vi "readCalib.vi"(8 "error in (no error) 2":errorcluster, 11 "Settings":T10={"CamSettings"={"Cam 0"={"position"=0.0, "pixelsize"=0.0, "start"=0.0, "end"=0.0, "center"=0.0, "Lens"=enum."FL1-f8x08", "Forward"=enum."off", "Spec_Calib_file 2"=path "Y:/100TWdata/ESMCalib/datFwd.txt", "map"=path "Y:/100TWdata/ESMCalib/mapFwd.txt", "y size"=0, "UserROI"={"Width"={"Value"=0.0, "Min"=0.0, "Max"=0.0, "StepSize"=0.0, "Tolerance"=0.0, "ValueActual"=0.0}, "Hight"={"Value"=0.0, "Min"=0.0, "Max"=0.0, "StepSize"=0.0, "Tolerance"=0.0, "ValueActual"=0.0}, "OffsetX"={"Value"=0.0, "Min"=0.0, "Max"=0.0, "StepSize"=0.0, "Tolerance"=0.0, "ValueActual"=0.0}, "OffsetY"={"Value"=0.0, "Min"=0.0, "Max"=0.0, "StepSize"=0.0, "Tolerance"=0.0, "ValueActual"=0.0}}, "CamMaxPixel"={"X"=0, "Y"=0}, "CamROI"={"Width"=0.0, "Hight"=0.0, "OffsetX"=0.0, "OffsetY"=0.0}}, "Cam 1"={"position"=0.0, "pixelsize"=0.0, "start"=0.0, "end"=0.0, "center"=0.0, "Lens"=enum."FL1-f8x08", "Forward"=enum."off", "Spec_Calib_file 2"=path "Y:/100TWdata/ESMCalib/datFwd.txt", "map"=path "Y:/100TWdata/ESMCalib/mapFwd.txt", "y size"=0, "UserROI"={"Width"={"Value"=0.0, "Min"=0.0, "Max"=0.0, "StepSize"=0.0, "Tolerance"=0.0, "ValueActual"=0.0}, "Hight"={"Value"=0.0, "Min"=0.0, "Max"=0.0, "StepSize"=0.0, "Tolerance"=0.0, "ValueActual"=0.0}, "OffsetX"={"Value"=0.0, "Min"=0.0, "Max"=0.0, "StepSize"=0.0, "Tolerance"=0.0, "ValueActual"=0.0}, "OffsetY"={"Value"=0.0, "Min"=0.0, "Max"=0.0, "StepSize"=0.0, "Tolerance"=0.0, "ValueActual"=0.0}}, "CamMaxPixel"={"X"=0, "Y"=0}, "CamROI"={"Width"=0.0, "Hight"=0.0, "OffsetX"=0.0, "OffsetY"=0.0}}, "Cam 2"={"position"=0.0, "pixelsize"=0.0, "start"=0.0, "end"=0.0, "center"=0.0, "Lens"=enum."FL1-f8x08", "Forward"=enum."off", "Spec_Calib_file 2"=path "Y:/100TWdata/ESMCalib/datFwd.txt", "map"=path "Y:/100TWdata/ESMCalib/mapFwd.txt", "y size"=0, "UserROI"={"Width"={"Value"=0.0, "Min"=0.0, "Max"=0.0, "StepSize"=0.0, "Tolerance"=0.0, "ValueActual"=0.0}, "Hight"={"Value"=0.0, "Min"=0.0, "Max"=0.0, "StepSize"=0.0, "Tolerance"=0.0, "ValueActual"=0.0}, "OffsetX"={"Value"=0.0, "Min"=0.0, "Max"=0.0, "StepSize"=0.0, "Tolerance"=0.0, "ValueActual"=0.0}, "OffsetY"={"Value"=0.0, "Min"=0.0, "Max"=0.0, "StepSize"=0.0, "Tolerance"=0.0, "ValueActual"=0.0}}, "CamMaxPixel"={"X"=0, "Y"=0}, "CamROI"={"Width"=0.0, "Hight"=0.0, "OffsetX"=0.0, "OffsetY"=0.0}}, "Cam 3"={"position"=0.0, "pixelsize"=0.0, "start"=0.0, "end"=0.0, "center"=0.0, "Lens"=enum."FL1-f8x08", "Forward"=enum."off", "Spec_Calib_file 2"=path "Y:/100TWdata/ESMCalib/datFwd.txt", "map"=path "Y:/100TWdata/ESMCalib/mapFwd.txt", "y size"=0, "UserROI"={"Width"={"Value"=0.0, "Min"=0.0, "Max"=0.0, "StepSize"=0.0, "Tolerance"=0.0, "ValueActual"=0.0}, "Hight"={"Value"=0.0, "Min"=0.0, "Max"=0.0, "StepSize"=0.0, "Tolerance"=0.0, "ValueActual"=0.0}, "OffsetX"={"Value"=0.0, "Min"=0.0, "Max"=0.0, "StepSize"=0.0, "Tolerance"=0.0, "ValueActual"=0.0}, "OffsetY"={"Value"=0.0, "Min"=0.0, "Max"=0.0, "StepSize"=0.0, "Tolerance"=0.0, "ValueActual"=0.0}}, "CamMaxPixel"={"X"=0, "Y"=0}, "CamROI"={"Width"=0.0, "Hight"=0.0, "OffsetX"=0.0, "OffsetY"=0.0}}}, "timeout"={"Value"=0.0, "Min"=0.0, "Max"=0.0, "StepSize"=0.0, "Tolerance"=0.0, "ValueActual"=0.0}, "Screws"={"Cam 0"={"S 0"={"0"=0, "1"=0, "2"=0, "3"=0}, "S 1"={"0"=0, "1"=0, "2"=0, "3"=0}, "S 2"={"0"=0, "1"=0, "2"=0, "3"=0}, "S 3"={"0"=0, "1"=0, "2"=0, "3"=0}, "S 4"={"0"=0, "1"=0, "2"=0, "3"=0}, "S 5"={"0"=0, "1"=0, "2"=0, "3"=0}}, "Cam 1"={"S 0"={"0"=0, "1"=0, "2"=0, "3"=0}, "S 1"={"0"=0, "1"=0, "2"=0, "3"=0}, "S 2"={"0"=0, "1"=0, "2"=0, "3"=0}, "S 3"={"0"=0, "1"=0, "2"=0, "3"=0}, "S 4"={"0"=0, "1"=0, "2"=0, "3"=0}, "S 5"={"0"=0, "1"=0, "2"=0, "3"=0}}, "Cam 2"={"S 0"={"0"=0, "1"=0, "2"=0, "3"=0}, "S 1"={"0"=0, "1"=0, "2"=0, "3"=0}, "S 2"={"0"=0, "1"=0, "2"=0, "3"=0}, "S 3"={"0"=0, "1"=0, "2"=0, "3"=0}, "S 4"={"0"=0, "1"=0, "2"=0, "3"=0}, "S 5"={"0"=0, "1"=0, "2"=0, "3"=0}}, "Cam 3"={"S 0"={"0"=0, "1"=0, "2"=0, "3"=0}, "S 1"={"0"=0, "1"=0, "2"=0, "3"=0}, "S 2"={"0"=0, "1"=0, "2"=0, "3"=0}, "S 3"={"0"=0, "1"=0, "2"=0, "3"=0}, "S 4"={"0"=0, "1"=0, "2"=0, "3"=0}, "S 5"={"0"=0, "1"=0, "2"=0, "3"=0}}}, "number of cam"=0.0, "X size"=0.0, "srewstart"={"Cam 0"=0.0, "Cam 1"=0.0, "Cam 2"=0.0, "Cam 3"=0.0}, "Save"=enum."off", "offset"=0.0, "localsavingpath"=path "", "ROIString"="", "exposure"={"Value"=0.0, "Min"=0.0, "Max"=0.0, "StepSize"=0.0, "Tolerance"=0.0, "ValueActual"=0.0}, "trigger"=enum."off"}) -> (0 "error out":errorcluster, 2 "fileCalib":cluster{"[0]":T1, "[1]":T1, "[2]":T1, "[3]":T1}, 3 "CamCalib":cluster{"[0]":T2, "[1]":T2, "[2]":T2, "[3]":T2}={"[0]"={"incident ANGLE COMPENSATION"=[], "dp/B [MeV/C/B]"=[], "charge compensation"=[], "Momentum [MeV/C]"=[], "energyDependence Input"=[], "pixel angle (y)"=[], "dp [MeV/C/] "=[], "angle 2Dfor spectrumj"=[], "dp [MeV/C] 2D"=[], "charge compensation 2D"=[], "Screen&Camera 2"={"Screen Orientation"="Regular", "Screen angle"="Flat", "Lens"=enum."FL1-f8x08", "Calibration (mm/pix)"=1.0}, "ROI info"={"npix-X"=0, "npix-Y"=0, "Left [pix]"=0.0, "Top [pix]"=0.0}, "Y 2D full angle"=[], "calib pixel"={"y1(pixel)"=[], "y2(pixel)"=[], "dp/B [MeV/C/B] (pixel)"=[], "energyDependence Input(pixel)"=[], "bending angle [deg](pixel)"=[], "total path(pixel)"=[], "pixel angle (y)(pixel)"=[], "energy dependence (pixel)"=[], "charge compensation (pixel)"=[], "Momentum [MeV/C](pixel)"=[], "angular compensation(pixel)"=[]}, "2D"={"dp"=[], "chargeCompensation"=[], "angle"=[], "Momentum"=[]}, "UserROI"={"Width"=0.0, "Hight"=0.0, "OffsetX"=0.0, "OffsetY"=0.0}, "final"={"X"=[], "xi"=[], "delta momentum"=0.0, "Y"=[], "yi"=[], "angle (Y)"=[], "delta angle"=0.0, "scale delta angle"=0.0, "intraX"=0.0, "intraY"=0.0, "mask"=[]}, "B[T]"=0.0, "index"=0.0}, "[1]"={"incident ANGLE COMPENSATION"=[], "dp/B [MeV/C/B]"=[], "charge compensation"=[], "Momentum [MeV/C]"=[], "energyDependence Input"=[], "pixel angle (y)"=[], "dp [MeV/C/] "=[], "angle 2Dfor spectrumj"=[], "dp [MeV/C] 2D"=[], "charge compensation 2D"=[], "Screen&Camera 2"={"Screen Orientation"="Regular", "Screen angle"="Flat", "Lens"=enum."FL1-f8x08", "Calibration (mm/pix)"=1.0}, "ROI info"={"npix-X"=0, "npix-Y"=0, "Left [pix]"=0.0, "Top [pix]"=0.0}, "Y 2D full angle"=[], "calib pixel"={"y1(pixel)"=[], "y2(pixel)"=[], "dp/B [MeV/C/B] (pixel)"=[], "energyDependence Input(pixel)"=[], "bending angle [deg](pixel)"=[], "total path(pixel)"=[], "pixel angle (y)(pixel)"=[], "energy dependence (pixel)"=[], "charge compensation (pixel)"=[], "Momentum [MeV/C](pixel)"=[], "angular compensation(pixel)"=[]}, "2D"={"dp"=[], "chargeCompensation"=[], "angle"=[], "Momentum"=[]}, "UserROI"={"Width"=0.0, "Hight"=0.0, "OffsetX"=0.0, "OffsetY"=0.0}, "final"={"X"=[], "xi"=[], "delta momentum"=0.0, "Y"=[], "yi"=[], "angle (Y)"=[], "delta angle"=0.0, "scale delta angle"=0.0, "intraX"=0.0, "intraY"=0.0, "mask"=[]}, "B[T]"=0.0, "index"=0.0}, "[2]"={"incident ANGLE COMPENSATION"=[], "dp/B [MeV/C/B]"=[], "charge compensation"=[], "Momentum [MeV/C]"=[], "energyDependence Input"=[], "pixel angle (y)"=[], "dp [MeV/C/] "=[], "angle 2Dfor spectrumj"=[], "dp [MeV/C] 2D"=[], "charge compensation 2D"=[], "Screen&Camera 2"={"Screen Orientation"="Regular", "Screen angle"="Flat", "Lens"=enum."FL1-f8x08", "Calibration (mm/pix)"=1.0}, "ROI info"={"npix-X"=0, "npix-Y"=0, "Left [pix]"=0.0, "Top [pix]"=0.0}, "Y 2D full angle"=[], "calib pixel"={"y1(pixel)"=[], "y2(pixel)"=[], "dp/B [MeV/C/B] (pixel)"=[], "energyDependence Input(pixel)"=[], "bending angle [deg](pixel)"=[], "total path(pixel)"=[], "pixel angle (y)(pixel)"=[], "energy dependence (pixel)"=[], "charge compensation (pixel)"=[], "Momentum [MeV/C](pixel)"=[], "angular compensation(pixel)"=[]}, "2D"={"dp"=[], "chargeCompensation"=[], "angle"=[], "Momentum"=[]}, "UserROI"={"Width"=0.0, "Hight"=0.0, "OffsetX"=0.0, "OffsetY"=0.0}, "final"={"X"=[], "xi"=[], "delta momentum"=0.0, "Y"=[], "yi"=[], "angle (Y)"=[], "delta angle"=0.0, "scale delta angle"=0.0, "intraX"=0.0, "intraY"=0.0, "mask"=[]}, "B[T]"=0.0, "index"=0.0}, "[3]"={"incident ANGLE COMPENSATION"=[], "dp/B [MeV/C/B]"=[], "charge compensation"=[], "Momentum [MeV/C]"=[], "energyDependence Input"=[], "pixel angle (y)"=[], "dp [MeV/C/] "=[], "angle 2Dfor spectrumj"=[], "dp [MeV/C] 2D"=[], "charge compensation 2D"=[], "Screen&Camera 2"={"Screen Orientation"="Regular", "Screen angle"="Flat", "Lens"=enum."FL1-f8x08", "Calibration (mm/pix)"=1.0}, "ROI info"={"npix-X"=0, "npix-Y"=0, "Left [pix]"=0.0, "Top [pix]"=0.0}, "Y 2D full angle"=[], "calib pixel"={"y1(pixel)"=[], "y2(pixel)"=[], "dp/B [MeV/C/B] (pixel)"=[], "energyDependence Input(pixel)"=[], "bending angle [deg](pixel)"=[], "total path(pixel)"=[], "pixel angle (y)(pixel)"=[], "energy dependence (pixel)"=[], "charge compensation (pixel)"=[], "Momentum [MeV/C](pixel)"=[], "angular compensation(pixel)"=[]}, "2D"={"dp"=[], "chargeCompensation"=[], "angle"=[], "Momentum"=[]}, "UserROI"={"Width"=0.0, "Hight"=0.0, "OffsetX"=0.0, "OffsetY"=0.0}, "final"={"X"=[], "xi"=[], "delta momentum"=0.0, "Y"=[], "yi"=[], "angle (Y)"=[], "delta angle"=0.0, "scale delta angle"=0.0, "intraX"=0.0, "intraY"=0.0, "mask"=[]}, "B[T]"=0.0, "index"=0.0}})   [LabVIEW 2020, in "MagAnalysis_Online.lvclass"]
uses:
  MagAnalysis_Online.lvclass
  MagAnalysis_Online/settings_TypDef.ctl
  CamSettings_Typdef.ctl
  CamSettingSUB_TypDEf.ctl
  CamAndObj_TypDEf.ctl
  OnOffTypeDef.ctl
  userROI.ctl
  source/Device Drivers/shared/numericVariable_TypeDef.ctl
  CamRoiTypDef.ctl
  SrewMaster_TYpDef.ctl
  srew_TypDEf.ctl
  ScrewSub_Typdef.ctl
  screwstart.ctl
  calib_Sub_Typdef.ctl
  ScreenCam2_TypDEf.ctl
  ROIInfo_TypDef.ctl
  calibPixel.ctl
  2DTypDef.ctl
  finalCalibTypdef.ctl
  configTypDEf.ctl
  specClustercommandTypdef.ctl
  source/Device Drivers/BaseDriver/BaseDriver.lvclass
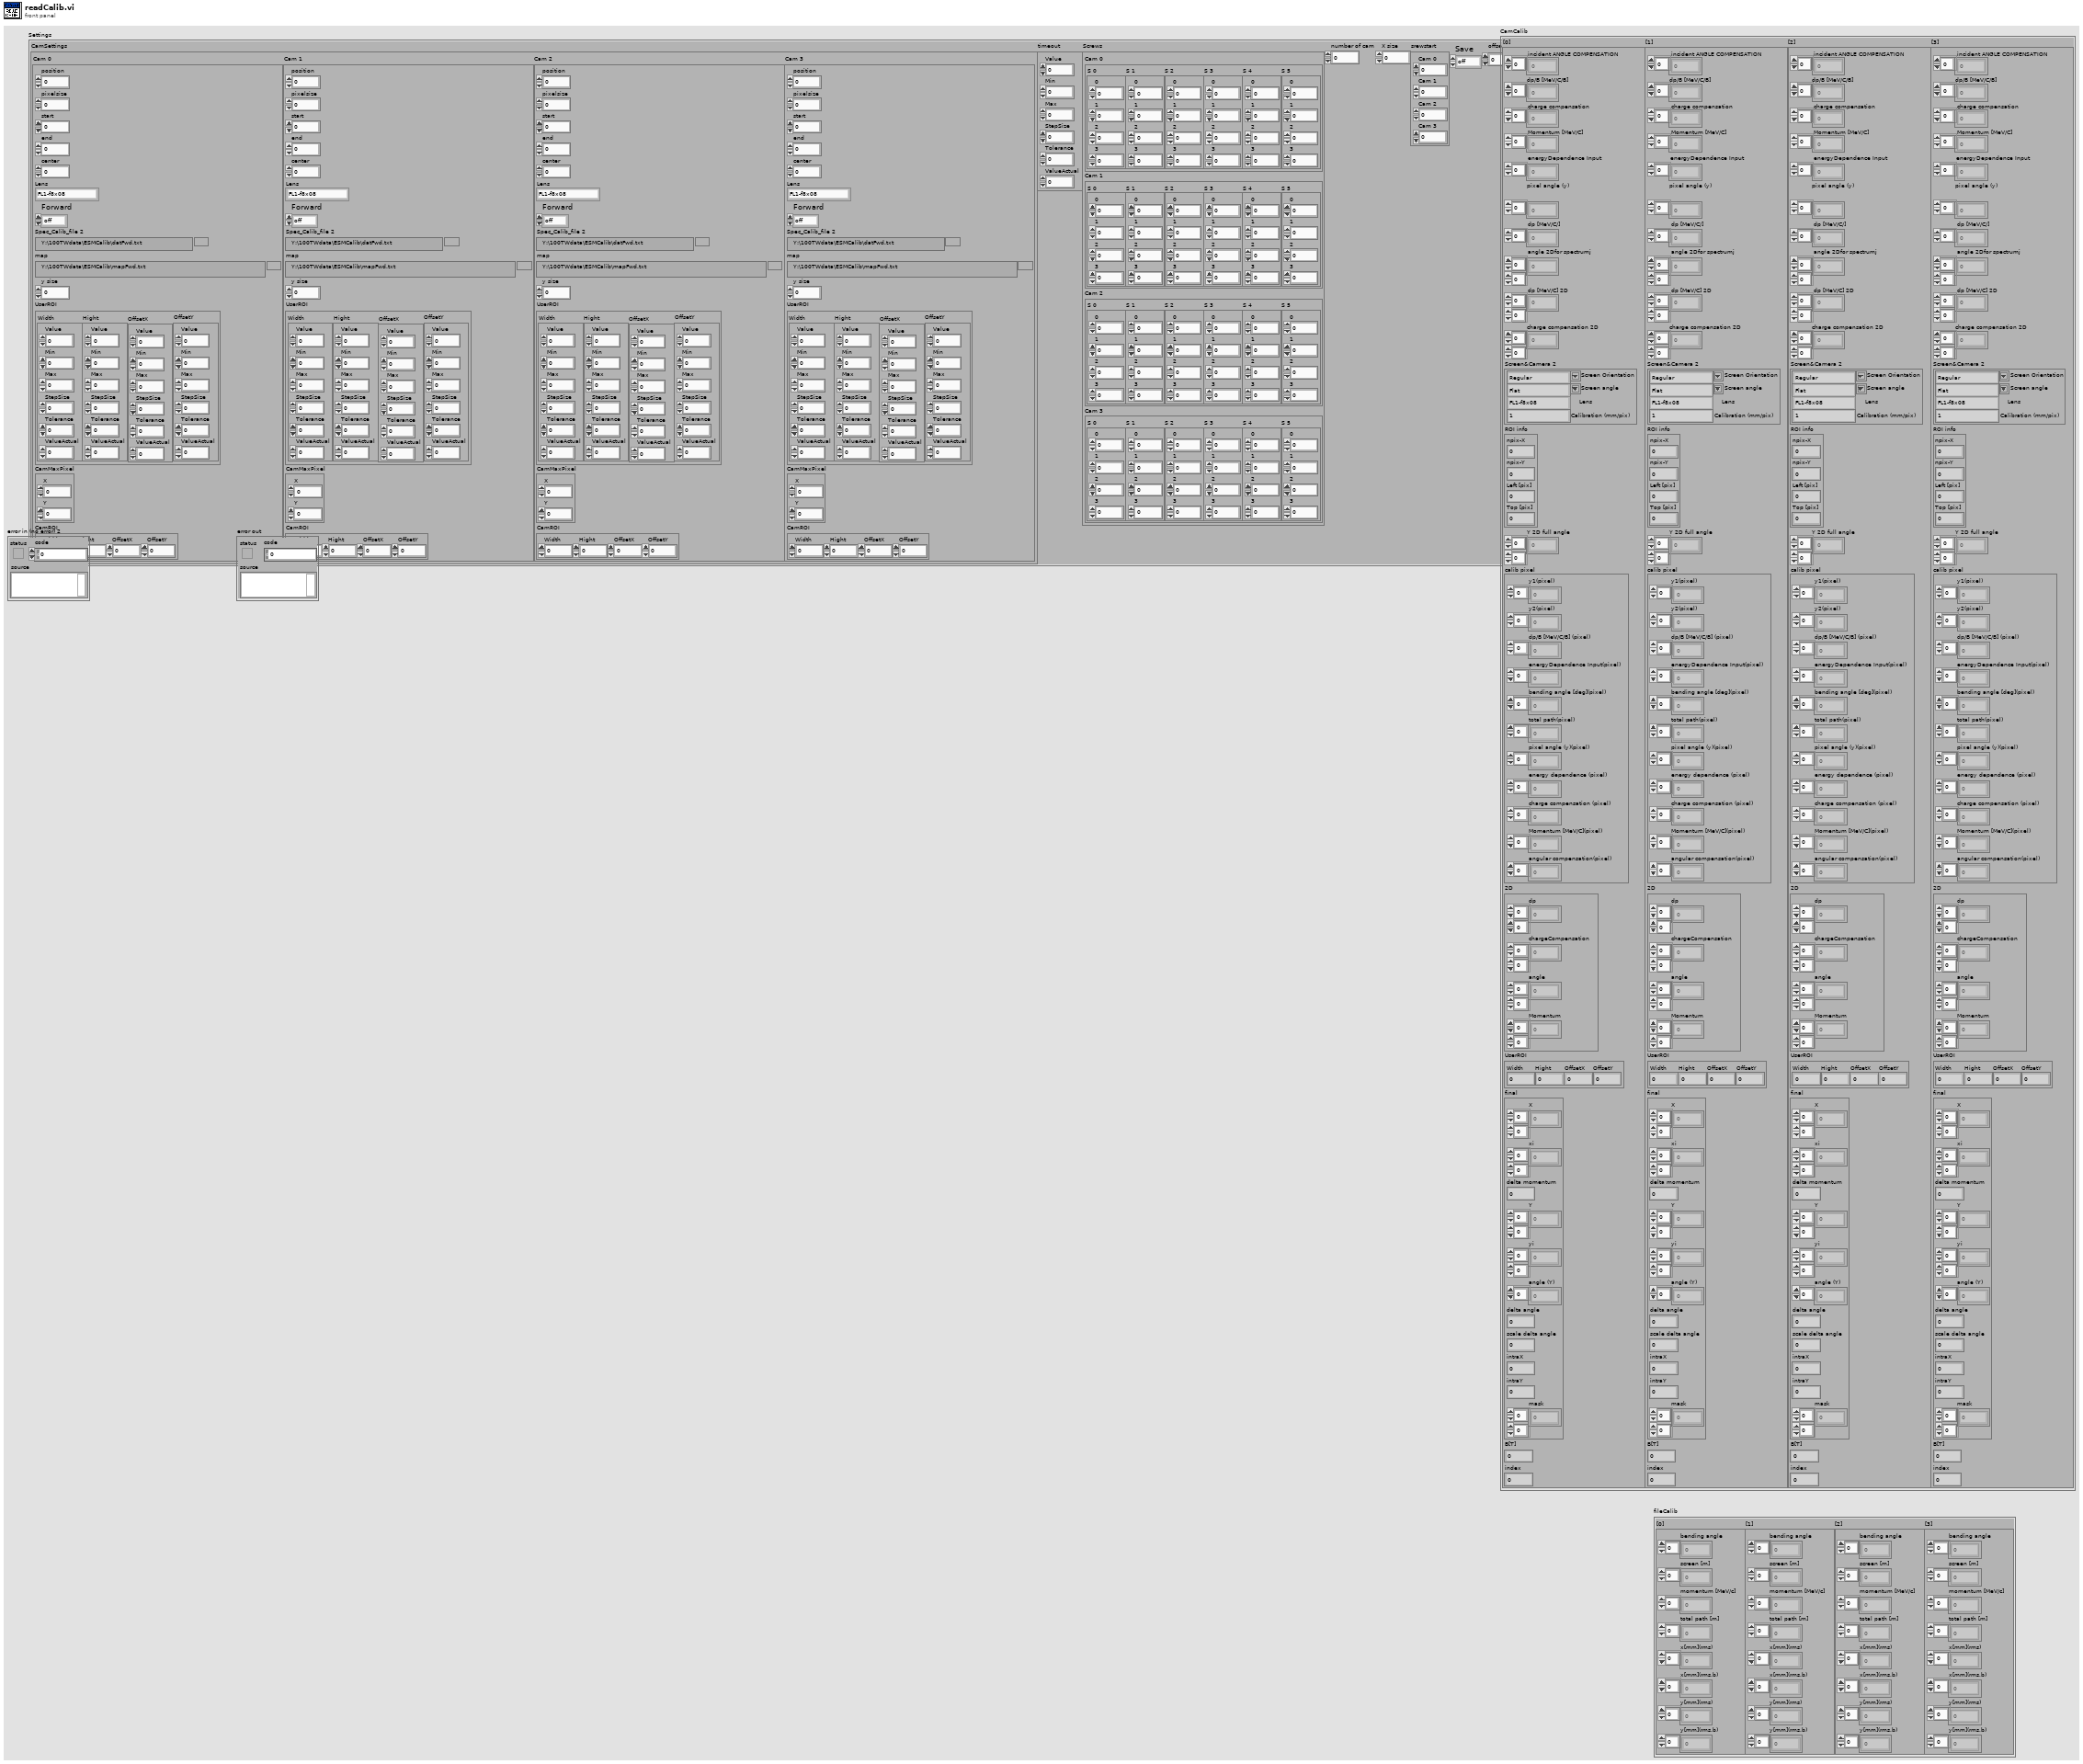
[diagram p1: front panel]
types:
  T1 = typedef "configTypDEf.ctl" = cluster{"bending angle":dbl[], "screen [m]":dbl[], "momentum [MeV/c]":dbl[], "total path [m]":dbl[], "x[mm](rms)":dbl[], "x[mm](rms,b)":dbl[], "y[mm](rms)":dbl[], "y[mm](rms,b)":dbl[]}
  T2 = typedef "calib_Sub_Typdef.ctl" = cluster{"incident ANGLE COMPENSATION":dbl[], "dp/B [MeV/C/B]":dbl[], "charge compensation":dbl[], "Momentum [MeV/C]":dbl[], "energyDependence Input":dbl[], "pixel angle (y)":dbl[], "dp [MeV/C/] ":dbl[], "angle 2Dfor spectrumj":dbl[][], "dp [MeV/C] 2D":dbl[][], "charge compensation 2D":dbl[][], "Screen&Camera 2":T3, "ROI info":T5, "Y 2D full angle":dbl[][], "calib pixel":T6, "2D":T7, "UserROI":T8, "final":T9, "B[T]":dbl, "index":dbl}
  T3 = typedef "ScreenCam2_TypDEf.ctl" = cluster{"Screen Orientation":string, "Screen angle":string, "Lens":T4, "Calibration (mm/pix)":dbl}
  T4 = typedef "CamAndObj_TypDEf.ctl" = enum16{"FL1-f8x08", "FL1-f8x06", "FL1-f8", "ch300-f50", "FL2G-f8", "FL3M14-f8", "FL3M14-f8x08", "FL3M14-f8x08(2x2)"}
  T5 = typedef "ROIInfo_TypDef.ctl" = cluster{"npix-X":i32, "npix-Y":i32, "Left [pix]":dbl, "Top [pix]":dbl}
  T6 = typedef "calibPixel.ctl" = cluster{"y1(pixel)":dbl[], "y2(pixel)":dbl[], "dp/B [MeV/C/B] (pixel)":dbl[], "energyDependence Input(pixel)":dbl[], "bending angle [deg](pixel)":dbl[], "total path(pixel)":dbl[], "pixel angle (y)(pixel)":dbl[], "energy dependence (pixel)":dbl[], "charge compensation (pixel)":dbl[], "Momentum [MeV/C](pixel)":dbl[], "angular compensation(pixel)":dbl[]}
  T7 = typedef "2DTypDef.ctl" = cluster{"dp":dbl[][], "chargeCompensation":dbl[][], "angle":dbl[][], "Momentum":dbl[][]}
  T8 = typedef "CamRoiTypDef.ctl" = cluster{"Width":dbl, "Hight":dbl, "OffsetX":dbl, "OffsetY":dbl}
  T9 = typedef "finalCalibTypdef.ctl" = cluster{"X":dbl[][], "xi":dbl[][], "delta momentum":dbl, "Y":dbl[][], "yi":dbl[][], "angle (Y)":dbl[], "delta angle":dbl, "scale delta angle":dbl, "intraX":dbl, "intraY":dbl, "mask":dbl[][]}
  T10 = typedef "MagAnalysis_Online.lvclass/settings_TypDef.ctl" = cluster{"CamSettings":T11, "timeout":T15, "Screws":T16, "number of cam":dbl, "X size":dbl, "srewstart":T19, "Save":T13, "offset":dbl, "localsavingpath":path, "ROIString":string, "exposure":T15, "trigger":T13}
  T11 = typedef "CamSettings_Typdef.ctl" = cluster{"Cam 0":T12, "Cam 1":T12, "Cam 2":T12, "Cam 3":T12}
  T12 = typedef "CamSettingSUB_TypDEf.ctl" = cluster{"position":dbl, "pixelsize":dbl, "start":dbl, "end":dbl, "center":dbl, "Lens":T4, "Forward":T13, "Spec_Calib_file 2":path, "map":path, "y size":i32, "UserROI":T14, "CamMaxPixel":cluster{"X":i32, "Y":i32}, "CamROI":T8}
  T13 = typedef "OnOffTypeDef.ctl" = enum16{"off", "on"}
  T14 = typedef "userROI.ctl" = cluster{"Width":T15, "Hight":T15, "OffsetX":T15, "OffsetY":T15}
  T15 = typedef "BaseDriver.lvclass/numericVariable_TypeDef.ctl" = cluster{"Value":dbl, "Min":dbl, "Max":dbl, "StepSize":dbl, "Tolerance":dbl, "ValueActual":dbl}
  T16 = typedef "SrewMaster_TYpDef.ctl" = cluster{"Cam 0":T17, "Cam 1":T17, "Cam 2":T17, "Cam 3":T17}
  T17 = typedef "srew_TypDEf.ctl" = cluster{"S 0":T18, "S 1":T18, "S 2":T18, "S 3":T18, "S 4":T18, "S 5":T18}
  T18 = typedef "ScrewSub_Typdef.ctl" = cluster{"0":i32, "1":i32, "2":i32, "3":i32}
  T19 = typedef "screwstart.ctl" = cluster{"Cam 0":dbl, "Cam 1":dbl, "Cam 2":dbl, "Cam 3":dbl}
  T20 = typedef "specClustercommandTypdef.ctl" = enum16{"init", "addCluster", "read", "clear"}
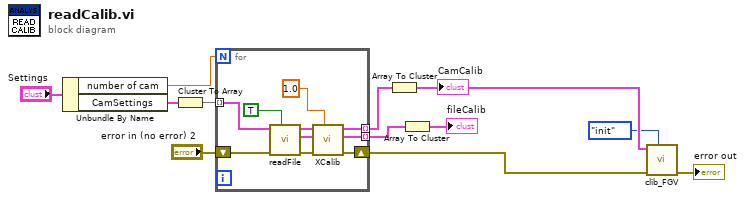
[diagram p0: block diagram]
diagram:
  n1 = Unbundle By Name("Settings") -> ("number of cam"=w8:dbl, "CamSettings"=w12:T11)
  n2 = Cluster To Array(cluster=w12) -> (array=w11:T12[])
  n3 = for {
    N: w8 -> [_]
    tunnel: w11 -> [w14] mode=indexing
    tunnel: [w15] -> w9 mode=indexing
    shift-right: [w16] -> w7
    shift-left: "error in (no error) 2" -> [w17]
    tunnel: [w13] -> w4 mode=indexing
    n4 = call "readFile.vi"("New (one file)"=TRUE, "error in (no error)"=w17, "Cam 1"=w14) -> ("error out"=w19:errorcluster, "Cluster"=w22:T1, "Cam 0"=w21:T12)  [unwired: 6 in]
    n5 = call "XCalib.vi"("B [T]"=1.0, "error in (no error)"=w19, "fileCalib"=w22, "DB calib"=w21) -> ("error out"=w16:errorcluster, "fileCalib out"=w13:T1, "cam calib"=w15:T2)  [unwired: 5 in]
  }
  n6 = Array To Cluster(array=w9) -> (cluster=w10:cluster{"[0]":T2, "[1]":T2, "[2]":T2, "[3]":T2})
  "CamCalib" <- w10
  n7 = Array To Cluster(array=w4) -> (cluster=→"fileCalib":cluster{"[0]":T1, "[1]":T1, "[2]":T1, "[3]":T1})
  n8 = call "clib_FGV.vi"("command"=specClustercommandTypdef."init", "error in (no error)"=w7, "Clibration"=w10) -> ("error out"=→"error out":errorcluster)  [unwired: 7 in, 1 out]
